vi "ObtainMessageQueues.vi"(8 "entrée d'erreur (pas d'erreur)":errorcluster) -> (0 "sortie d'erreur":errorcluster, 3 "Message queue":refnum<queue>)   [LabVIEW 2017, in "MessageQueues.lvlib"]
doc: "VI permettant la création d'une Pile (Message Queue) de manière générique."
uses:
  MessageQueues.lvlib
  Message Cluster.ctl
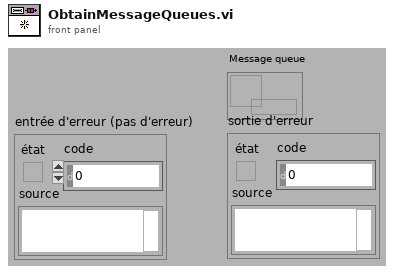
[diagram p1: front panel]
types:
  T1 = typedef "MessageQueues.lvlib/Message Cluster.ctl" = cluster{"Message":string, "Data":variant}
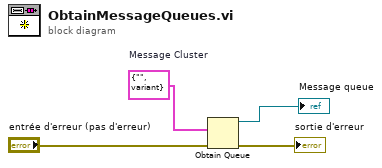
[diagram p0: block diagram]
diagram:
  w4 = T1 {"Message"="", "Data"=variant}  # Message Cluster
  n1 = Obtain Queue(element data type=w4, error in (no error)="entrée d'erreur (pas d'erreur)") -> (queue out=→"Message queue":refnum<queue>, error out=→"sortie d'erreur":errorcluster)  [unwired: 3 in, 1 out]
